vi "TangoAttributeChangeAndPeriodicEventTest.vi"() -> ()   [LabVIEW 2014, in "examples.lvlib"]
uses:
  vis/tango_vi.llb/_TangoSubscribeAttributeChangeEvent.vi
  vis/tango_vi.llb/_TangoSubscribeAttributePeriodicEvent.vi
  vis/tango_vi.llb/avToDoubleScalar.vi
  vis/tango_vi.llb/avToLongScalar.vi
  vis/tango_vi.llb/avToULongSpectrum.vi
  vis/tango_vi.llb/avToUShortSpectrum.vi
  examples.lvlib
  vis/tango_vi.llb/tango.lvlib
panel:
  out "Intensity Graph":u32[][](graph)
  out "Waveform Graph":u16[](graph)
  in  "events types":T1(array[ring])=[enum."PERIODIC_EVENT", enum."PERIODIC_EVENT"]
  in  "events sources":string[][](array[string])=[["sys/tg_test/1", "ushort_spectrum_ro"], ["sys/tg_test/1", "ulong_image_ro"]]
  out "Event Timeout":bool
  in  "timeout (ms)":i32=1000
  out "?":dbl(graph)=-95.9004706383706
  in  "Attribute name":string="long_scalar"
  out "?":i32(graph)=203
  out "Attribute Value":i32
  out "Event Timeout":bool
  in  "timeout (ms)":i32=1000
  in  "?":bool
  out "Attribute Value":dbl
  in  "Device Name":string="sys/tg_test/1"
  in  "Attribute Name":string="double_scalar"
  # "TANGO \"ATTRIBUTE EVENTS\" DEMO"
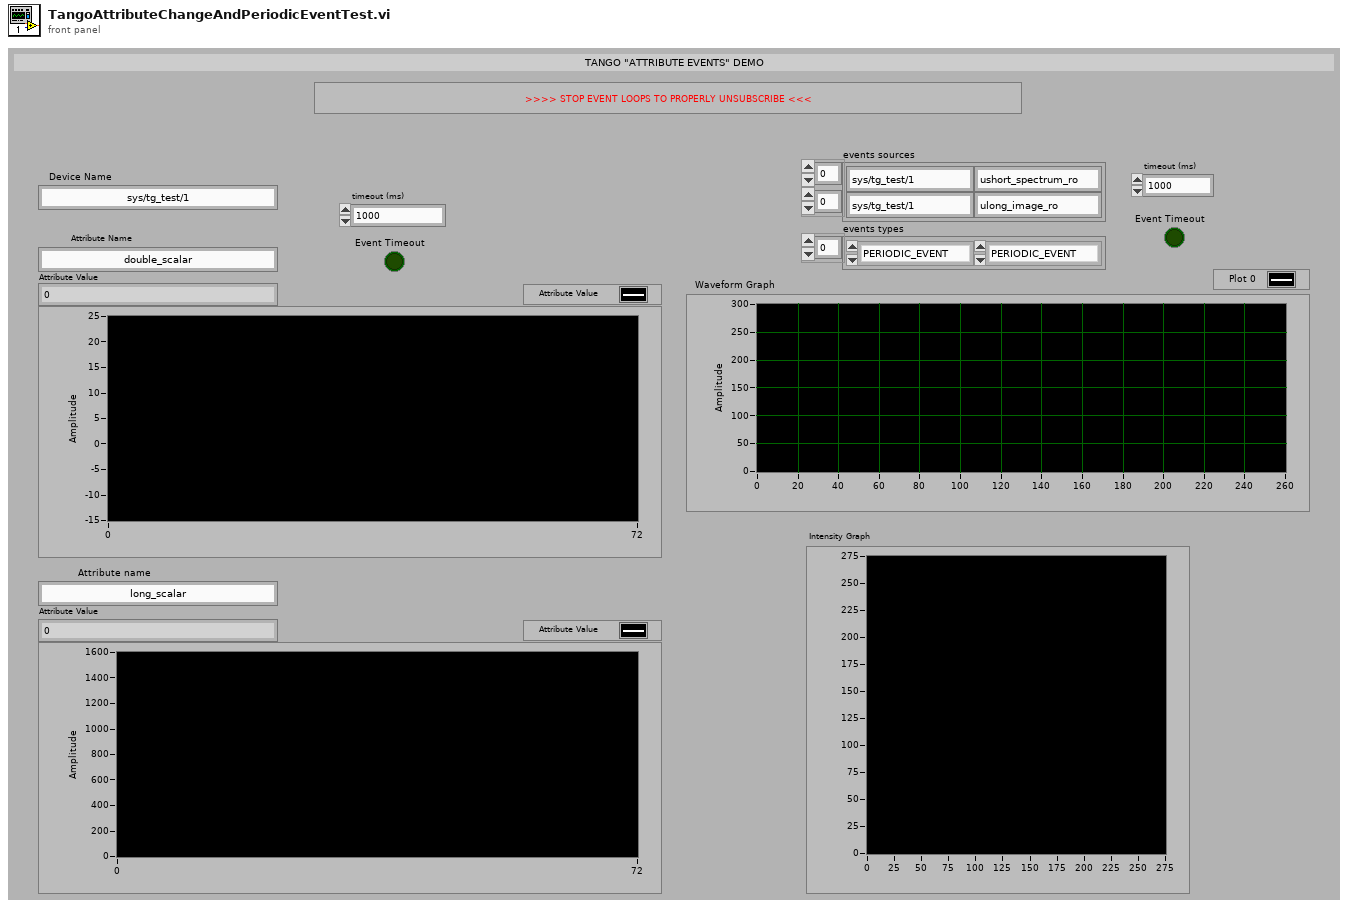
[diagram p1: front panel]
types:
  T1 = enum32{"CHANGE_EVENT", "DEPRECATED_QUALITY_EVENT", "PERIODIC_EVENT", "ARCHIVE_EVENT", "USER_EVENT", "ATTRIBUTE_CONF_EVENT", "DATA_READY_EVENT", "INTERFACE_CHANGE_EVENT", "UNKNOWN_EVENT"}[]
  T2 = typedef "tango.lvlib/_AttributeEventRef.ctl" = cluster{"user event ref":refnum<user-event>, "user event reg refnum":refnum<event-registration>}
  T3 = cluster{"device name":string, "attribute name":string, "quality value":i16, "quality string":string, "timestamp":dbl, "dim. x":i32, "dim. y":i32, "value":u8[], "error code":i32, "error stack":string[], "data type":u16}
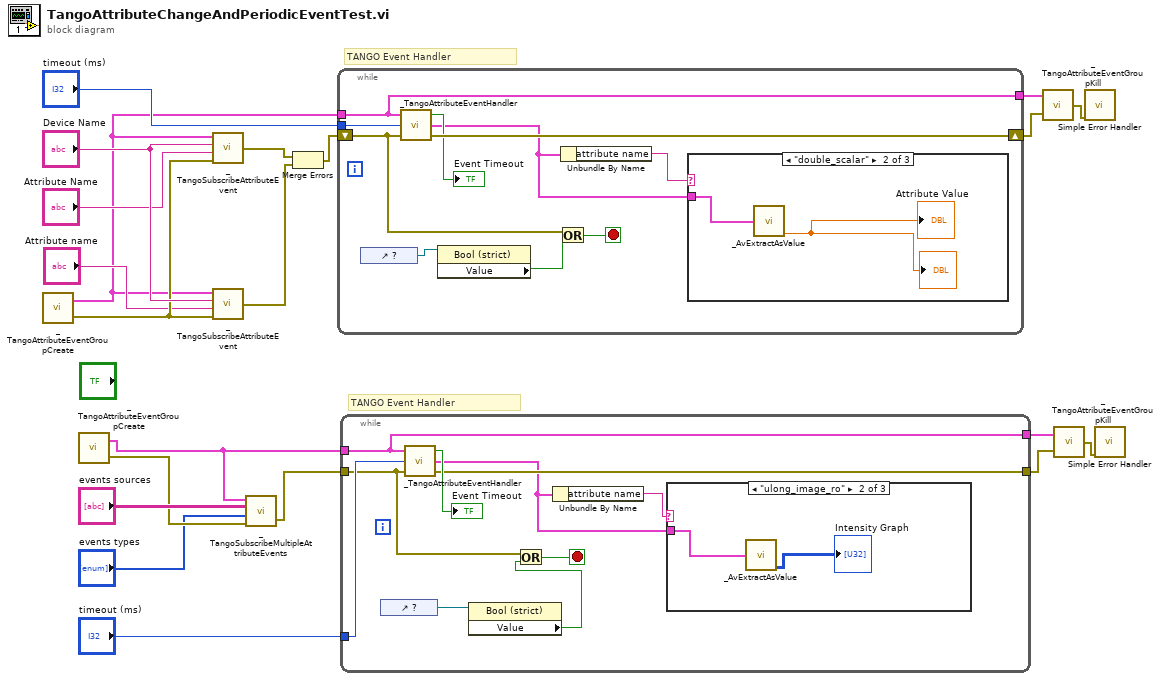
[diagram p0: block diagram]
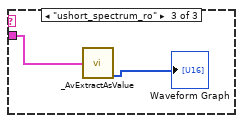
[diagram p3: hidden frame]
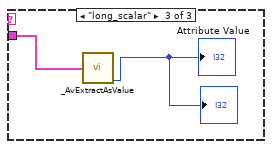
[diagram p5: hidden frame]
diagram:
  # "TANGO Event Handler"
  # "TANGO Event Handler"
  n1 = call "_TangoAttributeEventGroupCreate.vi"() -> ("attribute event ref."=w6:T2, "error out"=w14:errorcluster)  [unwired: 1 in]
  n2 = call "_TangoAttributeEventGroupCreate.vi"() -> ("attribute event ref."=w1:T2, "error out"=w12:errorcluster)  [unwired: 1 in]
  n3 = call-poly "_TangoSubscribeAttributeEvent.vi"("error in"=w14, "attribute name"="Attribute Name", "device name"="Device Name", "attribute event ref."=w6) -> ("error out"=w17:errorcluster)
  n4 = call-poly "_TangoSubscribeAttributeEvent.vi"("error in"=w14, "attribute name"="Attribute name", "device name"="Device Name", "attribute event ref."=w6) -> ("error out"=w16:errorcluster)
  n5 = call "_TangoSubscribeMultipleAttributeEvents.vi"("error in"=w12, "events types"="events types", "events sources"="events sources", "attribute event ref."=w1) -> ("error out"=w10:errorcluster)  [unwired: 1 out]
  n6 = Merge Errors(w17, w16) -> (w15:errorcluster)
  n7 = while {
    shift-right: [w30] -> w4
    shift-left: w15 -> [w23]
    tunnel: "timeout (ms)" -> [w28]
    tunnel: w6 -> [w25]
    tunnel: [w25] -> w5
    stop <- w22 stop-if-true
    n8 = control-ref of="?"() -> (w31:refnum<vi>)
    n9 = call "_TangoAttributeEventHandler.vi"("error in"=w23, "timeout (ms)"=w28, "attribute event ref."=w25) -> ("error out"=w30:errorcluster, "attribute raw data"=w26:T3, "event timeout"=→"Event Timeout":bool)
    n10 = property class="Bool (strict)"(reference=w31) -> ("Value"=w24:bool)  [unwired: 1 in, 2 out]
    n11 = Or(x=w23, y=w24) -> (x .or. y?=w22:bool)
    n12 = Unbundle By Name(w26) -> ("attribute name"=w29:string)
    n13 = case shown="\"double_scalar\"" w29 {
      tunnel: w26 -> [_ w32 w35]
      frame Default {
      }
      frame "double_scalar" {
        n14 = call-poly "_AvExtractAsValue.vi"("attribute value"=w32) -> ("value"=→"Attribute Value" →"?":dbl)  [unwired: 4 out]
      }
      frame "long_scalar" {
        n15 = call-poly "_AvExtractAsValue.vi"("attribute value"=w35) -> ("value"=→"Attribute Value" →"?":i32)  [unwired: 4 out]
      }
    }
  }
  n16 = while {
    tunnel: w10 -> [w38]
    tunnel: [w44] -> w2
    tunnel: "timeout (ms)" -> [w43]
    tunnel: w1 -> [w40]
    tunnel: [w40] -> w3
    stop <- w37 stop-if-true
    n17 = control-ref of="?"() -> (w39:refnum<vi>)
    n18 = call "_TangoAttributeEventHandler.vi"("error in"=w38, "timeout (ms)"=w43, "attribute event ref."=w40) -> ("error out"=w44:errorcluster, "attribute raw data"=w41:T3, "event timeout"=→"Event Timeout":bool)
    n19 = property class="Bool (strict)"(reference=w39) -> ("Value"=w36:bool)  [unwired: 1 in, 2 out]
    n20 = Or(x=w38, y=w36) -> (x .or. y?=w37:bool)
    n21 = Unbundle By Name(w41) -> ("attribute name"=w42:string)
    n22 = case shown="\"ulong_image_ro\"" w42 {
      tunnel: w41 -> [_ w47 w48]
      frame Default {
      }
      frame "ulong_image_ro" {
        n23 = call-poly "_AvExtractAsValue.vi"("attribute value"=w47) -> ("value"=→"Intensity Graph":u32[][])  [unwired: 4 out]
      }
      frame "ushort_spectrum_ro" {
        n24 = call-poly "_AvExtractAsValue.vi"("attribute value"=w48) -> ("value"=→"Waveform Graph":u16[])  [unwired: 4 out]
      }
    }
  }
  n25 = call "_TangoAttributeEventGroupKill.vi"("error in"=w4, "attribute event ref."=w5) -> ("error out"=w18:errorcluster)
  n26 = call "_TangoAttributeEventGroupKill.vi"("error in"=w2, "attribute event ref."=w3) -> ("error out"=w9:errorcluster)
  n27 = call <vilib>:"Simple Error Handler.vi"("error in (no error)"=w18) -> ()  [unwired: 4 in, 5 out]
  n28 = call <vilib>:"Simple Error Handler.vi"("error in (no error)"=w9) -> ()  [unwired: 4 in, 5 out]
